vi "dfd_Render Difference Equation.vi"(5 "fonts input":T2(array[cluster])=[{"Font Name:"="tahoma", "Size"=13, "Strikeout?"=FALSE, "Italic?"=FALSE, "Underline?"=FALSE, "Outline?"=TRUE, "Shadow?"=FALSE, "Bold?"=FALSE}, {"Font Name:"="tahoma", "Size"=13, "Strikeout?"=FALSE, "Italic?"=FALSE, "Underline?"=FALSE, "Outline?"=TRUE, "Shadow?"=FALSE, "Bold?"=FALSE}, {"Font Name:"="tahoma", "Size"=13, "Strikeout?"=FALSE, "Italic?"=FALSE, "Underline?"=FALSE, "Outline?"=TRUE, "Shadow?"=FALSE, "Bold?"=FALSE}], 6 "display format":u16(ring) items=["Feedback on left and feed forward on right", "Feedback and feed forward on right", "Feedback and feed forward on right in 1 line"], 7 "format string":string="%#.4g", 8 "error in":errorcluster, 9 "origin":cluster{"left":i16, "top":i16}, 10 "transfer function":cluster{"numerator":dbl[], "denominator":dbl[]}={"numerator"=[1.0, 2.0], "denominator"=[1.0, -1.0]}, 11 "picture in":picture) -> (0 "error out":errorcluster, 1 "size":cluster{"width":i16, "height":i16}, 3 "picture out":picture)   [LabVIEW 2017, in "NI_DigFilter_Process.lvlib"]
uses:
  <vilib>/addons/Digital Filter Design/NI_DigFilter_Process.lvlib
  <vilib>/Analysis/polynomials.llb/Remove Zero Coefficients (DBL).vi
  <vilib>/Analysis/NI_AALPro.lvlib
panel:
  in  "bracket":cluster{"left":string, "right":string}={"left"="[", "right"="]"}
  in  "variables":T1={"system output function"="y", "argument"="n", "system input function"="x"}
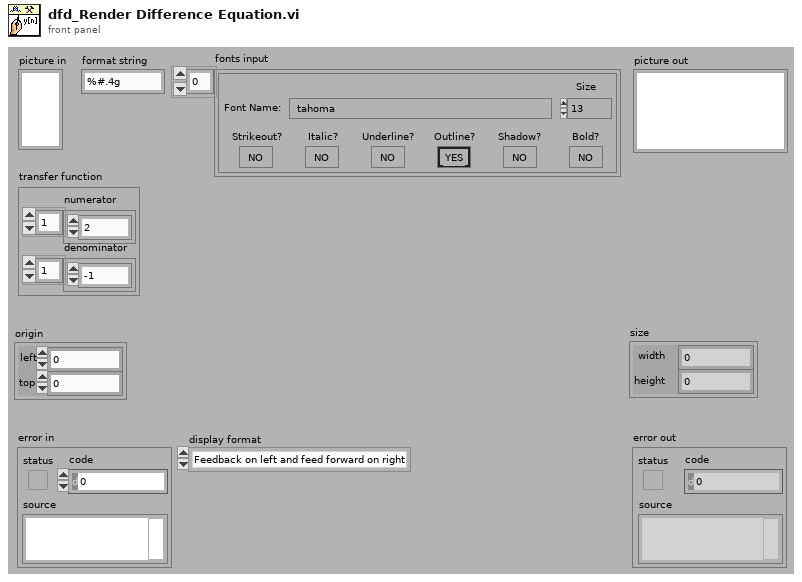
[diagram p1: front panel]
types:
  T1 = cluster{"system output function":string, "argument":string, "system input function":string}
  T2 = cluster{"Font Name:":string, "Size":i16, "Strikeout?":bool, "Italic?":bool, "Underline?":bool, "Outline?":bool, "Shadow?":bool, "Bold?":bool}[]
  T3 = cluster{"left":i16, "top":i16, "left":i16, "top":i16}
  T4 = cluster{"Font Name:":string, "Size":i16, "Strikeout?":bool, "Italic?":bool, "Underline?":bool, "Outline?":bool, "Shadow?":bool, "Bold?":bool}
  T5 = cluster{"system output function":string, "argument":string, "bracket":cluster{"left":string, "right":string}}
  T6 = cluster{"left":i16, "top":i16, "right":i16, "bottom":i16}
  T7 = cluster{"bottom":i16, "bottom":i16, "bottom":i16, "bottom":i16}
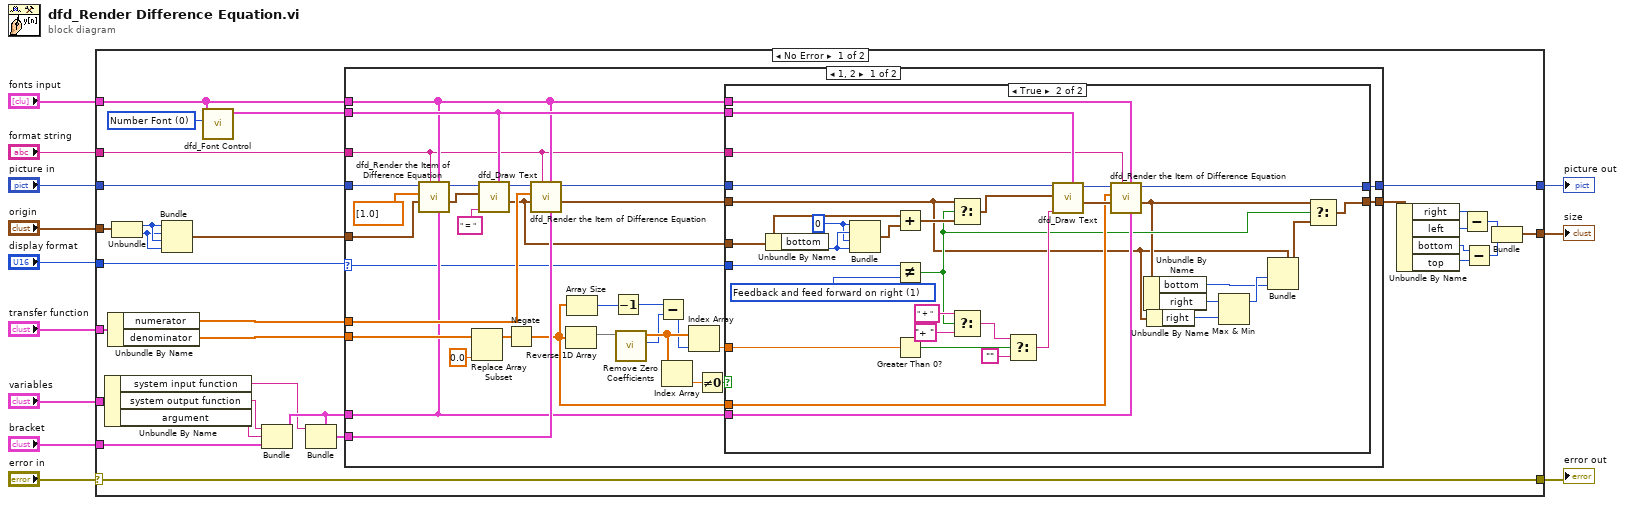
[diagram p0: block diagram]
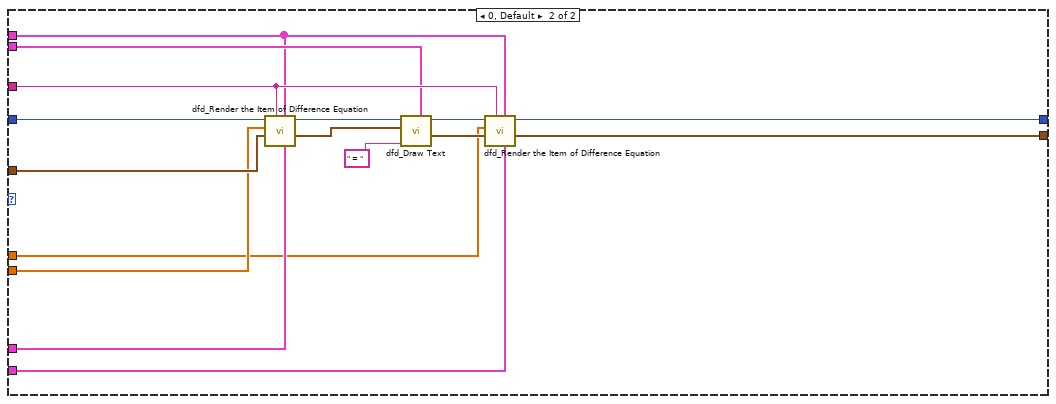
[diagram p3: hidden frame]
diagram:
  n1 = case shown="No Error" "error in" {
    selector: "error in" -> [w26 w126]
    tunnel: "origin" -> [w25 _]
    tunnel: "picture in" -> [w42 _]
    tunnel: [w14 _] -> w10
    tunnel: "format string" -> [w41 _]
    tunnel: [w40 _] -> w8
    tunnel: "transfer function" -> [w37 _]
    tunnel: "fonts input" -> [w34 _]
    tunnel: "variables" -> [w33 _]
    tunnel: "bracket" -> [w32 _]
    tunnel: [w26 w126] -> w2
    tunnel: "display format" -> [w13 _]
    frame No Error {
      w38 = u16 0 items=["Number Font", "Variable Font", "Script Font"] ("Tpye")
      n2 = Unbundle By Name(w33) -> ("system input function"=w27:string, "system output function"=w28:string, "argument"=w31:string)
      n3 = Unbundle By Name(w37) -> ("numerator"=w36:dbl[], "denominator"=w35:dbl[])
      n4 = Unbundle(w25) -> ("left"=w24:i16, "top"=w23:i16)
      n5 = Bundle("left"=w24, "top"=w23, "left"=w24, "top"=w23) -> (w22:T3)  [unwired: 1 out]
      n6 = call <vilib>:"dfd_Font Control.vi"("tpye"=w38, "fonts input"=w34) -> ("font output"=w39:T4)  [unwired: 9 out]
      n7 = Bundle("system output function"=w28, "argument"=w31, "bracket"=w32) -> (w29:T5)  [unwired: 1 out]
      n8 = Bundle(cluster=w29, "system output function"=w27) -> (w30:T5)  [unwired: 2 out]
      n9 = case shown="1, 2" w13 {
        selector: w13 -> [w54 _]
        tunnel: w42 -> [w74 w123]
        tunnel: w41 -> [w65 w120]
        tunnel: [w70 w119] -> w40
        tunnel: w39 -> [w69 w117]
        tunnel: w36 -> [w68 w110]
        tunnel: w35 -> [w62 w111]
        tunnel: w34 -> [w66 w116]
        tunnel: w30 -> [w63 w115]
        tunnel: w29 -> [w61 w114]
        tunnel: w22 -> [w67 w113]
        tunnel: [w64 w112] -> w21
        frame 1, 2 {
          n10 = call <vilib>:"dfd_Render the Item of Difference Equation.vi"("format control"=w61, "fonts input"=w66, "format string"=w65, "rect in"=w67, "coefficients array"=dbl[] [1.0] ("denominator"), "picture in"=w74) -> ("rect out"=w52:T6, "picture out"=w73:picture)  [unwired: 2 in, 2 out]
          n11 = Replace Array Subset(array=w62, new element=0.0 ("new element/subarray")) -> (w59:dbl[])  [unwired: 1 in]
          n12 = call <vilib>:"dfd_Draw Text.vi"("font input"=w69, "text"=" = ", "rect in"=w52, "picture in"=w73) -> ("rect out"=w50:T6, "picture out"=w72:picture)  [unwired: 4 in, 2 out]
          n13 = Negate(x=w59) -> (-x=w47:dbl[])
          n14 = call <vilib>:"dfd_Render the Item of Difference Equation.vi"("format control"=w63, "fonts input"=w66, "format string"=w65, "rect in"=w50, "coefficients array"=w68, "picture in"=w72) -> ("rect out"=w51:T6, "picture out"=w71:picture)  [unwired: 2 in, 2 out]
          n15 = Reverse 1D Array(array=w47) -> (reversed array=w60:dbl[])
          n16 = Array Size(array=w47) -> (size(s)=w44:i32)
          n17 = Decrement(x=w44) -> (x-1=w43:i32)
          n18 = call-poly <vilib>:"Remove Zero Coefficients.vi"("P(x) In"=w60) -> ("number of zero coefficients"=w46:i32, "P(x) Out"=w49:dbl[])  [unwired: 2 in, 7 out]
          n19 = Subtract(x=w43, y=w46) -> (x-y=w45:i32)
          n20 = Index Array(array=w49) -> (element=w48:dbl)  [unwired: 1 in]
          n21 = Index Array(array=w49, index=w45) -> (element=w57:dbl)
          n22 = Not Equal To 0?(x=w48) -> (x != 0?=w58:bool)
          n23 = case shown="True" w58 {
            tunnel: w71 -> [w76 w108]
            tunnel: [w76 w107] -> w70
            tunnel: w69 -> [_ w106]
            tunnel: w51 -> [w75 w82]
            tunnel: w66 -> [_ w105]
            tunnel: w65 -> [_ w104]
            tunnel: [w75 w85] -> w64
            tunnel: w61 -> [_ w102]
            tunnel: w47 -> [_ w101]
            tunnel: w57 -> [_ w100]
            tunnel: w50 -> [_ w83]
            tunnel: w54 -> [_ w92]
            frame False {
            }
            frame True {
              w77 = u16 1 items=["Feedback on left and feed forward on right", "Feedback and feed forward on right", "Feedback and feed forward on right in 1 line"] ("display format")
              w95 = i16 0 ("bottom")
              n24 = Unbundle By Name(w83) -> ("bottom"=w96:i16)
              n25 = Bundle("bottom"=w95, "bottom"=w96, "bottom"=w95, "bottom"=w96) -> (w91:T7)  [unwired: 1 out]
              n26 = Add(x=w83, y=w91) -> (x+y=w93:cluster{i16, i16, i16, "bottom":i16})
              n27 = Not Equal?(x=w92, y=w77) -> (x != y?=w87:bool)
              n28 = Greater Than 0?(x=w100) -> (x > 0?=w99:bool)
              n29 = Select(t=w82, s=w87, f=w93) -> (s? t:f=w94:T6)
              n30 = Select(t=" + ", s=w87, f="+ ") -> (s? t:f=w90:string)
              n31 = Select(t=w90, s=w99, f="") -> (s? t:f=w98:string)
              n32 = call <vilib>:"dfd_Draw Text.vi"("font input"=w106, "text"=w98, "rect in"=w94, "picture in"=w108) -> ("rect out"=w103:T6, "picture out"=w109:picture)  [unwired: 4 in, 2 out]
              n33 = call <vilib>:"dfd_Render the Item of Difference Equation.vi"("format control"=w102, "fonts input"=w105, "format string"=w104, "rect in"=w103, "coefficients array"=w101, "picture in"=w109) -> ("rect out"=w86:T6, "picture out"=w107:picture)  [unwired: 2 in, 2 out]
              n34 = Unbundle By Name(w86) -> ("bottom"=w78:i16, "right"=w81:i16)
              n35 = Unbundle By Name(w82) -> ("right"=w80:i16)
              n36 = Max & Min(x=w81, y=w80) -> (max(x,y)=w79:i16)  [unwired: 1 out]
              n37 = Bundle(cluster=w82, "right"=w79, "bottom"=w78) -> (w84:T6)  [unwired: 2 out]
              n38 = Select(t=w86, s=w87, f=w84) -> (s? t:f=w85:T6)
            }
          }
        }
        frame 0, Default {
          n39 = call <vilib>:"dfd_Render the Item of Difference Equation.vi"("format control"=w114, "fonts input"=w116, "format string"=w120, "rect in"=w113, "coefficients array"=w111, "picture in"=w123) -> ("rect out"=w122:T6, "picture out"=w124:picture)  [unwired: 2 in, 2 out]
          n40 = call <vilib>:"dfd_Draw Text.vi"("font input"=w117, "text"=" = ", "rect in"=w122, "picture in"=w124) -> ("rect out"=w121:T6, "picture out"=w125:picture)  [unwired: 4 in, 2 out]
          n41 = call <vilib>:"dfd_Render the Item of Difference Equation.vi"("format control"=w115, "fonts input"=w116, "format string"=w120, "rect in"=w121, "coefficients array"=w110, "picture in"=w125) -> ("rect out"=w112:T6, "picture out"=w119:picture)  [unwired: 2 in, 2 out]
        }
      }
      n42 = Unbundle By Name(w21) -> ("right"=w20:i16, "left"=w19:i16, "bottom"=w18:i16, "top"=w17:i16)
      n43 = Subtract(x=w20, y=w19) -> (x-y=w16:i16)
      n44 = Subtract(x=w18, y=w17) -> (x-y=w15:i16)
      n45 = Bundle(w16, w15) -> (w14:cluster{i16, i16})  [unwired: 1 out]
    }
    frame Error {
    }
  }
  "size" <- w10
  "picture out" <- w8
  "error out" <- w2
